vi "set_field.vi"(8 "phi":dbl, 9 "theta (xy-ebene)":dbl, 10 "Magnitude (mT)":dbl, 11 "VISA-Ressourcenname":refnum<visa-resource-name>="COM7") -> ()   [LabVIEW 2011]
panel:
  out "source 4":dbl
  out "source 3":dbl
  out "source 2":dbl
  out "source 1":dbl
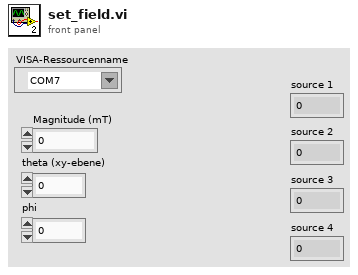
[diagram p1: front panel]
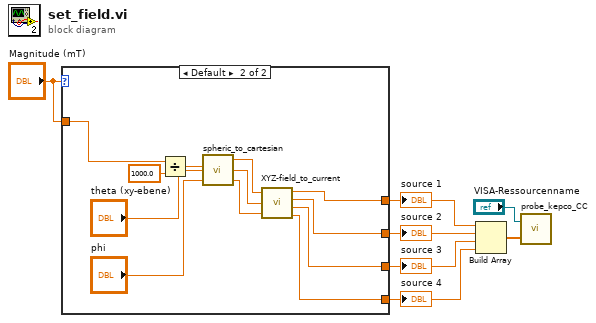
[diagram p0: block diagram]
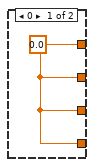
[diagram p2: hidden frame]
diagram:
  n1 = case shown="Default" "Magnitude (mT)" {
    tunnel: "Magnitude (mT)" -> [_ w15]
    tunnel: [w8 w14] -> w4
    tunnel: [w8 w13] -> w3
    tunnel: [w8 w12] -> w2
    tunnel: [w8 w11] -> w1
    frame 0 {
      w8 = 0.0 ("current 1")
    }
    frame Default {
      n2 = Divide(x=w15, y=1000.0) -> (x/y=w19:dbl)
      n3 = call "spheric_to_cartesian.vi"("phi"="phi", "theta (xy-ebene)"="theta (xy-ebene)", "Magnitude (T)"=w19) -> ("Z"=w9:dbl, "Y"=w10:dbl, "X"=w18:dbl)
      n4 = call "XYZ-field_to_current.vi"("X"=w18, "Y"=w10, "Z"=w9) -> ("current 1"=w14:dbl, "current 2"=w11:dbl, "current 3"=w12:dbl, "current 4"=w13:dbl)
    }
  }
  "source 1" <- w4
  "source 2" <- w1
  "source 3" <- w2
  "source 4" <- w3
  n5 = Build Array(w4, w1, w2, w3) -> (w6:dbl[])
  n6 = call "probe_kepco_CC.vi"("strommatrix"=w6, "VISA-Ressourcenname"="VISA-Ressourcenname") -> ()  [unwired: 1 out]
